vi "whole_setup_control_RT_v1229.vi"() -> ()   [LabVIEW 2021]
uses:
  <vilib>/Utility/file.llb/Read Delimited Spreadsheet (DBL).vi
  <vilib>/FPGAPlugInAG/cRIO-9038/niLvFpga_Open_cRIO-9038.vi
  <vilib>/rvi/interface/common/dynamic/niFpgaDynamicAddResources.vi
  <vilib>/FPGAPlugInAG/Dynamic/niLvFpga_Abort_Dynamic.vi
  <vilib>/FPGAPlugInAG/Dynamic/niLvFpga_Run_Dynamic.vi
  <vilib>/Utility/error.llb/Error Cluster From Error Code.vi
  <vilib>/rvi/errors/niLvFpgaAdjustHostInterfaceError.vi
  <vilib>/Utility/file.llb/Write Delimited Spreadsheet (DBL).vi
  <vilib>/FPGAPlugInAG/Dynamic/niLvFpga_Close_Dynamic.vi
  <vilib>/rvi/interface/nirviOpenFPGA/nirviOpenFPGA.xnode
  FPGA Bitfiles/voltagescopemain_FPGATarget_wholesetupcontro_vB3ODMckxO8.lvbitx
  whole_setup_control_FPGA_v1229.vi
  <vilib>/rvi/interface/nirviMethod/nirviMethod.xnode
  <vilib>/rvi/interface/nirviReadWriteControl/nirviReadWriteControl.xnode
  <vilib>/rvi/interface/nirviCloseFPGA/nirviCloseFPGA.xnode
  <vilib>/rvi/errors/niLvFpgaMergeErrorWithErrorCode.vi
  NiFpgaLv.dll
  <vilib>/rvi/interface/Simulation/niFpgaSimulationCallBeginRW.vi
  <vilib>/FPGAPlugInAG/Dynamic/niLvFpga_StopFifo_Dynamic.vi
  <vilib>/FPGAPlugInAG/Dynamic/niLvFpga_StartFifo_Dynamic.vi
  <vilib>/FPGAPlugInAG/Dynamic/niLvFpga_WriteFifo_Dynamic.vi
  <vilib>/FPGAPlugInAG/Dynamic/niLvFpga_ReadFifo_Dynamic.vi
panel:
  out "Numeric":i32=9
  in  "Signal array length 2":u32=1245
  in  "debug laser delay offset":i32=698
  in  "real laser pulse time (x4us)":i32=10
  in  "laser trigger start points":u32[](array[numeric])=[19, 61, 104, 140, 173, 215, 259, 331, 366, 401, 443, 487, 527, 605, 648, 693, 735, 767, 801, 841, 877, 954, 988, 1021, 1061, 1110, 1153, 1188, 1222, 565]
  in  "update laser triggers RT":bool
  in  "laser ON":bool
  out "Cycle us spent":dbl=4980.0
  in  "Signal array length":u32=1245
  in  "write galvo signal to":path=path "/home/lvuser/zgwang/20231229_4980us_output_signal_corr.dat"
  in  "Write galvo singal to txt RT":bool
  in  "DO 4 laser trigger delay":i32=698
  in  "DO 3 camera trigger delay - DO 4 laser trigger delay":i32=5
  in  "trigger debug?":bool
  in  "debugging and behavior \ncamera trigger delay (loops)":i32
  in  "3F0 freq X":i32=3
  in  "2F0 freq X":i32=5
  in  "camera trigger ON":bool
  in  "Galvo1 corr delay - laser delay":i32=545
  in  "G1 corr amplitude":fxp<+/-,32,16>
  in  "Galvo1 delay":i32=589
  out "ticks spent update":u32=65
  in  "update galvo drive signal RT":bool
  in  "laser delay increament":i32=10
  out "laser delay disp (loops)":i32=1878
  in  "laser delay":i32=118
  out "Loop ticks spent":u32=120
  in  "laser exposure (loops)":i32=10
  in  "Piezo offset":sgl=5.0
  in  "Piezo mag":sgl=2.58
  in  "2F0 amplitude":sgl=0.00255
  in  "3F0 amplitude":sgl=0.0858
  in  "2F0 phase":i32=792
  in  "3F0 phase":i32=555
  in  "Galvo1 offset (mV)":sgl=-448.0
  in  "Galvo1 mag (mV)":sgl=1.0
  out "all rows":dbl[][](array[numeric])
  in  "start output":bool=TRUE
  out "Data transfer finished":bool=TRUE
  in  "output data #":i32=1245
  in  "output loop ticks":u32=160
  in  "stop":bool
  out "array length":i32=1245
  out "Empty Elements Remaining":u32=15139
  out "loop N":i32=10
  in  "file path (dialog if empty)":path=path "/home/lvuser/zgwang/20231229_4980us_output_signal.dat"
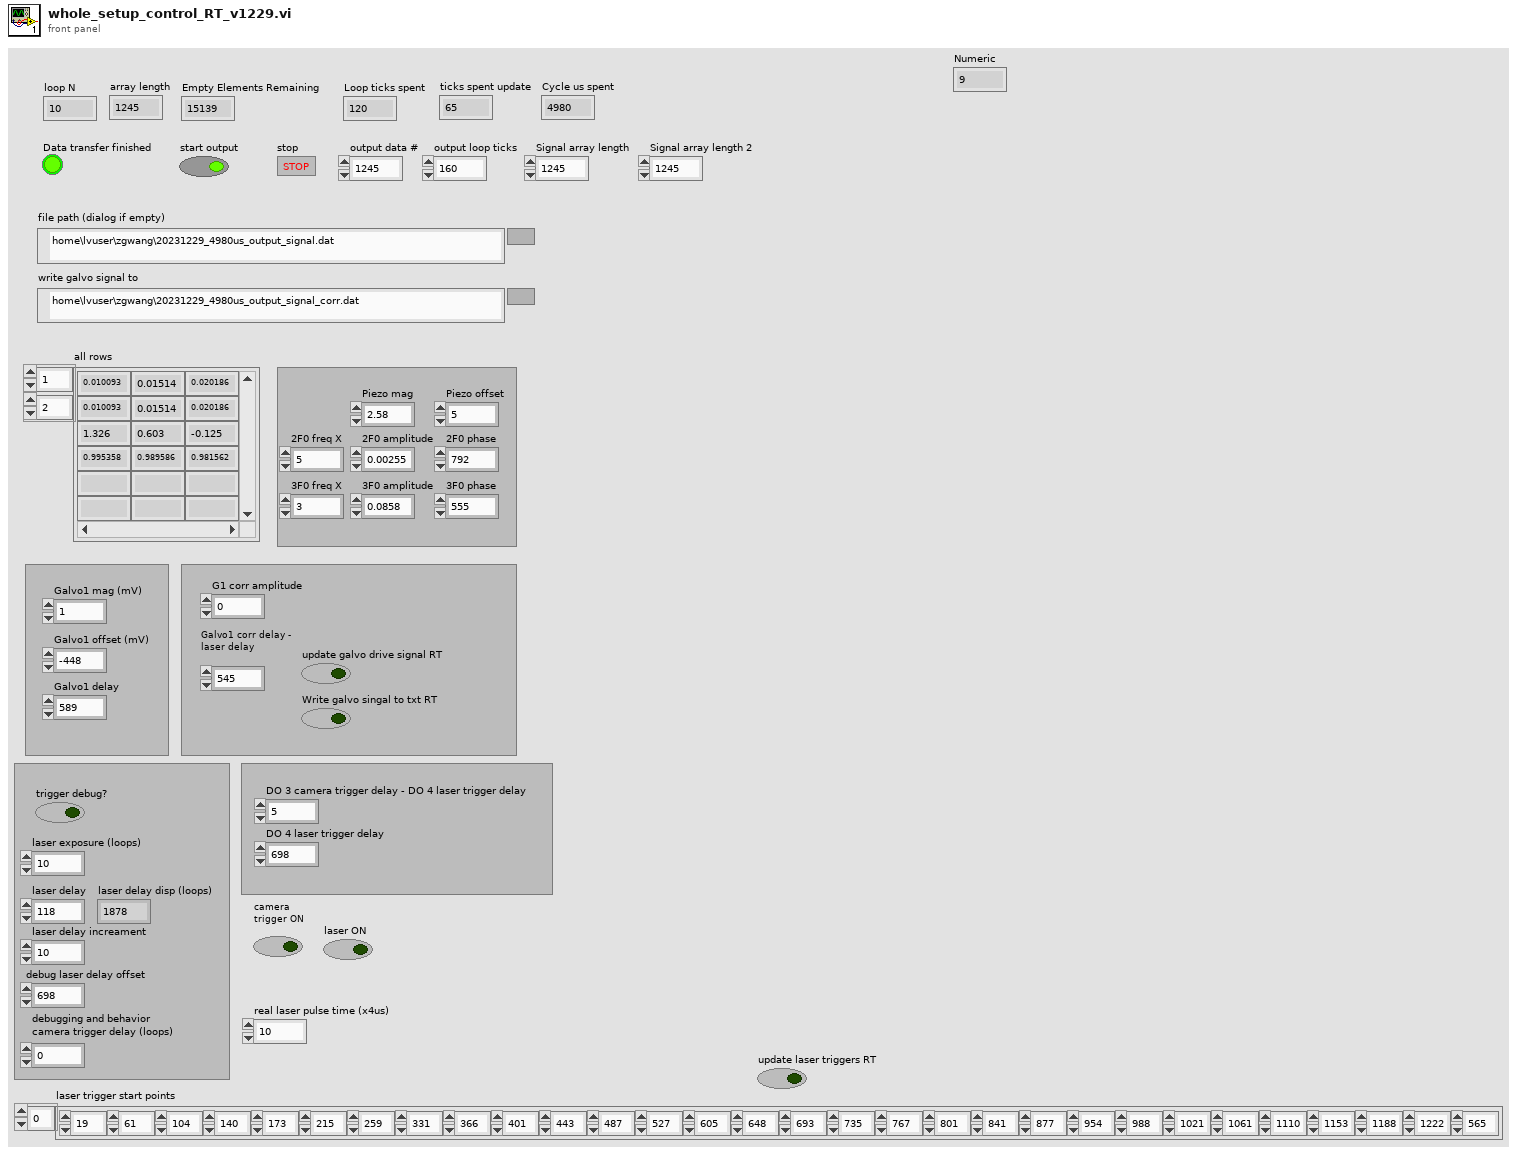
[diagram p1: front panel]
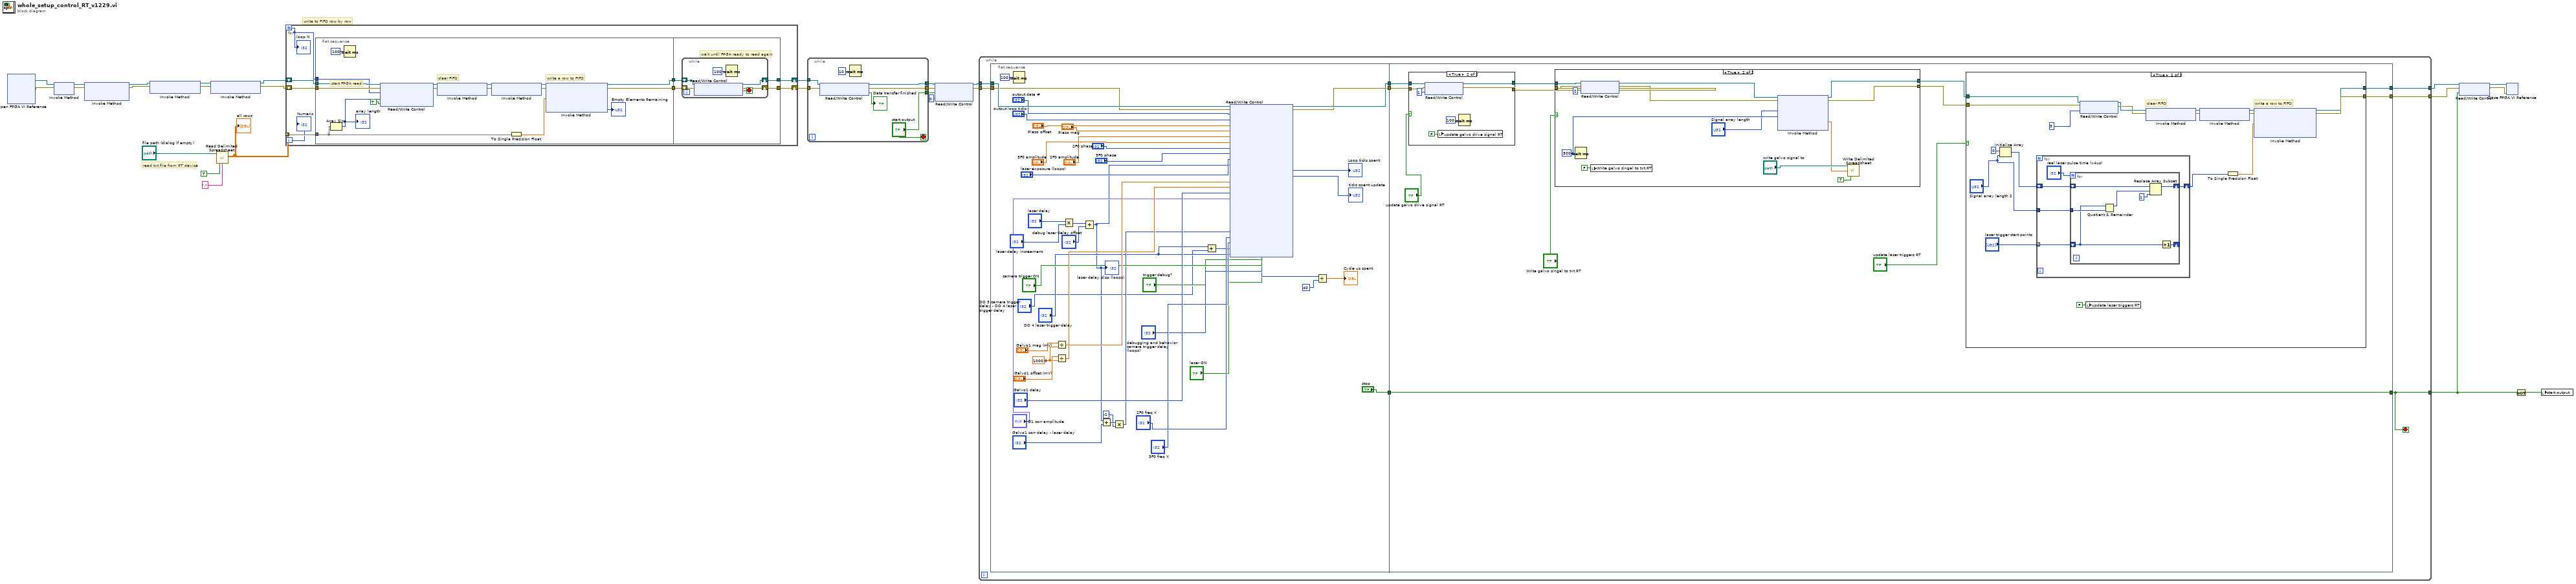
[diagram p0: block diagram]
diagram:
  # "write to FIFO row by row"
  # "read txt file from RT device"
  n1 = xnode "Open FPGA VI Reference"() -> ("FPGA VI Reference Out"=w17:refnum<k20>, "error out"=w14:errorcluster)  [unwired: 2 in]
  n2 = xnode "Invoke Method"("FPGA VI Reference In"=w17, "error in"=w14) -> ("FPGA VI Reference Out"=w16:refnum<k20>, "error out"=w15:errorcluster)
  n3 = xnode "Invoke Method"("FPGA VI Reference In"=w16, "error in"=w15) -> ("FPGA VI Reference Out"=w9:refnum<k20>, "error out"=w8:errorcluster)  [unwired: 1 in]
  n4 = xnode "Invoke Method"("FPGA VI Reference In"=w9, "error in"=w8) -> ("FPGA VI Reference Out"=w11:refnum<k20>, "error out"=w10:errorcluster)
  n5 = xnode "Invoke Method"("FPGA VI Reference In"=w11, "error in"=w10) -> ("FPGA VI Reference Out"=w7:refnum<k20>, "error out"=w6:errorcluster)
  n6 = call-poly <vilib>:"Read Delimited Spreadsheet.vi"("file path (dialog if empty)"="file path (dialog if empty)", "transpose? (F)"=TRUE, "delimiter (\\t)"="," ("delimiter (\\t)")) -> ("all rows"=w25:dbl[][])  [unwired: 7 in, 5 out]
  "all rows" <- w25
  n7 = for {
    N -> [w32]
    tunnel: w25 -> [w37] mode=indexing
    shift-right: [w31] -> w19
    shift-left: w7 -> [w35]
    shift-right: [w30] -> w18
    shift-left: w6 -> [w36]
    i -> [w29]
    n8 = flat-sequence {
      tunnel: w37 -> [w45]
      tunnel: w36 -> [w53]
      tunnel: w35 -> [w52]
      tunnel: [w51] -> w34
      tunnel: [w49] -> w33
      tunnel: w32 -> [w47]
      tunnel: w34 -> [w58]
      tunnel: w33 -> [w57]
      tunnel: [w56] -> w31
      tunnel: [w55] -> w30
      frame #0 {
        # "clear FIFO"
        # "write a row to FIFO"
        # "start FPGA read"
        n9 = Array Size(array=w45) -> (size(s)=w54:i32)
        "array length" <- w54
        n10 = Wait (ms)(milliseconds to wait=u32 100) -> ()  [unwired: 1 out]
        n11 = xnode "Read/Write Control"("FPGA VI Reference In"=w52, "error in"=w53, "data row #"=w47, "array length"=w54, "FPGA start to read FIFO"=TRUE) -> ("FPGA VI Reference Out"=w41:refnum<k20>, "error out"=w40:errorcluster)
        n12 = xnode "Invoke Method"("FPGA VI Reference In"=w41, "error in"=w40) -> ("FPGA VI Reference Out"=w43:refnum<k20>, "error out"=w42:errorcluster)
        n13 = xnode "Invoke Method"("FPGA VI Reference In"=w43, "error in"=w42) -> ("FPGA VI Reference Out"=w39:refnum<k20>, "error out"=w38:errorcluster)
        n14 = To Single Precision Float(number=w45) -> (single precision float=w44:sgl[])
        n15 = xnode "Invoke Method"("FPGA VI Reference In"=w39, "error in"=w38, "Data"=w44) -> ("FPGA VI Reference Out"=w51:refnum<k20>, "error out"=w49:errorcluster, "Empty Elements Remaining"=→"Empty Elements Remaining":u32)  [unwired: 1 in]
      }
      frame #1 {
        # "wait until FPGA ready to read again"
        n16 = while {
          shift-right: [w60] -> w56
          shift-left: w58 -> [w62]
          shift-right: [w59] -> w55
          shift-left: w57 -> [w61]
          stop <- w64 stop-if-true
          n17 = xnode "Read/Write Control"("FPGA VI Reference In"=w62, "error in"=w61) -> ("FPGA VI Reference Out"=w60:refnum<k20>, "error out"=w59:errorcluster, "FPGA finish read row"=w64:bool)
          n18 = Wait (ms)(milliseconds to wait=u32 100) -> ()  [unwired: 1 out]
        }
      }
    }
    "loop N" <- w32
    "Numeric" <- w29
  }
  n19 = while {
    tunnel: ["start output"] -> w24
    tunnel: [w67] -> w21
    tunnel: [w66] -> w20
    tunnel: w19 -> [w69]
    tunnel: w18 -> [w68]
    stop <- "start output" stop-if-true
    n20 = xnode "Read/Write Control"("FPGA VI Reference In"=w69, "error in"=w68) -> ("FPGA VI Reference Out"=w67:refnum<k20>, "error out"=w66:errorcluster, "Data transfer finished"=→"Data transfer finished":bool)
    n21 = Wait (ms)(milliseconds to wait=u32 10) -> ()  [unwired: 1 out]
  }
  n22 = xnode "Read/Write Control"("FPGA VI Reference In"=w21, "error in"=w20, "start output"=w24, "FPGA loop case"=u32 0) -> ("FPGA VI Reference Out"=w23:refnum<k20>, "error out"=w22:errorcluster)
  n23 = while {
    tunnel: w23 -> [w79]
    tunnel: w22 -> [w78]
    tunnel: [w77] -> w12
    tunnel: [w73] -> w2
    tunnel: [w72] -> w1
    stop <- w77 stop-if-true
    n24 = flat-sequence {
      tunnel: w79 -> [w123]
      tunnel: w78 -> [w122]
      tunnel: [w121] -> w76
      tunnel: [w120] -> w75
      tunnel: ["stop"] -> w74
      tunnel: [w136] -> w77
      tunnel: w74 -> [w136]
      tunnel: w75 -> [w131]
      tunnel: w76 -> [w132]
      tunnel: [w126] -> w73
      tunnel: [w125] -> w72
      frame #0 {
        w108 = sgl 1000.0 ("y")
        n25 = Wait (ms)(milliseconds to wait=u32 100) -> ()  [unwired: 1 out]
        n26 = Divide(x="Galvo1 mag (mV)", y=w108) -> (x/y=w103:sgl)
        n27 = Divide(x="Galvo1 offset (mV)", y=w108) -> (x/y=w102:sgl)
        n28 = Multiply(x="laser delay", y="laser delay increament") -> (x*y=w82:i32)
        n29 = Add(x=w82, y="debug laser delay offset") -> (x+y=w80:i32)
        "laser delay disp (loops)" <- w80
        n30 = Add(x=w80, y="Galvo1 corr delay - laser delay") -> (x+y=w99:i32)
        n31 = Multiply(x=w99, y=-1) -> (x*y=w92:i32)
        n32 = Add(x="DO 4 laser trigger delay", y="DO 3 camera trigger delay - DO 4 laser trigger delay") -> (x+y=w83:i32)
        n33 = xnode "Read/Write Control"("FPGA VI Reference In"=w123, "error in"=w122, "output data #"="output data #", "output loop ticks"="output loop ticks", "Piezo offset"="Piezo offset", "Piezo mag"="Piezo mag", "2F0 amplitude"="2F0 amplitude", "3F0 amplitude"="3F0 amplitude", "2F0 phase relative to F0"="2F0 phase", "3F0 phase relative to F0"="3F0 phase", "laser exposure (loops)"="laser exposure (loops)", "laser delay (loops)"=w80, "Galvo1 mag"=w103, "Galvo1 offset"=w102, "Galvo1 delay"="Galvo1 delay", "G1 corr amplitude"="G1 corr amplitude", "Galvo1 corr delay"=w92, "2F0 freq X"="2F0 freq X", "3F0 freq X"="3F0 freq X", "DO 3 delay"=w83, "DO 4 delay"="DO 4 laser trigger delay", "trigger debug?"="trigger debug?", "camera trigger ON"="camera trigger ON", "camera trigger delay (loops)"="debugging and behavior \ncamera trigger delay (loops)", "laser ON"="laser ON") -> ("FPGA VI Reference Out"=w121:refnum<k20>, "error out"=w120:errorcluster, "Loop ticks spent"=→"Loop ticks spent":u32, "ticks spent update"=→"ticks spent update":u32, "Cycle tick spent"=w89:u32)
        n34 = Divide(x=w89, y=u32 40) -> (x/y=→"Cycle us spent":dbl)
      }
      frame #1 {
        n35 = case shown="True" "update galvo drive signal RT" {
          tunnel: w132 -> [w169 w177]
          tunnel: [w169 w176] -> w134
          tunnel: [w170 w175] -> w133
          tunnel: w131 -> [w170 w174]
          frame False {
          }
          frame True {
            n36 = xnode "Read/Write Control"("FPGA VI Reference In"=w177, "error in"=w174, "FPGA loop case"=u32 1) -> ("FPGA VI Reference Out"=w176:refnum<k20>, "error out"=w175:errorcluster)
            n37 = local write "update galvo drive signal RT"(FALSE ("update galvo drive signal RT")) -> ()
            n38 = Wait (ms)(milliseconds to wait=u32 100) -> ()  [unwired: 1 out]
          }
        }
        n39 = case shown="True" "Write galvo singal to txt RT" {
          tunnel: w134 -> [w179 w192]
          tunnel: w133 -> [w178 w191]
          tunnel: [w179 w186] -> w128
          tunnel: [w178 w185] -> w127
          frame False {
          }
          frame True {
            w184 = u32 500 ("milliseconds to wait")
            n40 = Wait (ms)(milliseconds to wait=w184) -> ()  [unwired: 1 out]
            n41 = xnode "Read/Write Control"("FPGA VI Reference In"=w192, "error in"=w191, "FPGA loop case"=u32 2) -> ("FPGA VI Reference Out"=w188:refnum<k20>, "error out"=w187:errorcluster)
            n42 = local write "Write galvo singal to txt RT"(FALSE ("Write galvo singal to txt RT")) -> ()
            n43 = xnode "Invoke Method"("FPGA VI Reference In"=w188, "error in"=w187, "Number of Elements"="Signal array length", "Timeout (ms)"=w184) -> ("FPGA VI Reference Out"=w186:refnum<k20>, "error out"=w185:errorcluster, "Data"=w182:sgl[])  [unwired: 1 out]
            n44 = call-poly <vilib>:"Write Delimited Spreadsheet.vi"("file path (dialog if empty)"="write galvo signal to", "1D data"=w182, "transpose? (no:F)"=TRUE) -> ()  [unwired: 11 in, 2 out]
          }
        }
        n45 = case shown="True" "update laser triggers RT" {
          tunnel: w128 -> [w137 w144]
          tunnel: w127 -> [w138 w142]
          tunnel: [w138 w147] -> w125
          tunnel: [w137 w146] -> w126
          frame False {
          }
          frame True {
            # "clear FIFO"
            # "write a row to FIFO"
            n46 = Initialize Array(u32 0 ("element"), "Signal array length 2") -> (w154:u32[])
            n47 = for {
              tunnel: "laser trigger start points" -> [w160] mode=indexing
              shift-right: [w159] -> w148
              shift-left: w154 -> [w161]
              tunnel: "Signal array length 2" -> [w157]
              n48 = for {
                N: "real laser pulse time (x4us)" -> [_]
                shift-right: [w165] -> w159
                shift-left: w161 -> [w168]
                shift-right: [w166] -> _
                shift-left: w160 -> [w163]
                tunnel: w157 -> [w164]
                n49 = Quotient & Remainder(x=w163, y=w164) -> (x-y*floor(x/y)=w162:u32)  [unwired: 1 out]
                n50 = Replace Array Subset(array=w168, new element=u32 1 ("new element/subarray"), index=w162) -> (w165:u32[])
                n51 = Increment(x=w163) -> (x+1=w166:u32)
              }
            }
            n52 = xnode "Read/Write Control"("FPGA VI Reference In"=w144, "error in"=w142, "FPGA loop case"=u32 3) -> ("FPGA VI Reference Out"=w143:refnum<k20>, "error out"=w141:errorcluster)
            n53 = local write "update laser triggers RT"(FALSE ("update laser triggers RT")) -> ()
            n54 = xnode "Invoke Method"("FPGA VI Reference In"=w143, "error in"=w141) -> ("FPGA VI Reference Out"=w153:refnum<k20>, "error out"=w152:errorcluster)
            n55 = xnode "Invoke Method"("FPGA VI Reference In"=w153, "error in"=w152) -> ("FPGA VI Reference Out"=w151:refnum<k20>, "error out"=w150:errorcluster)
            n56 = To Single Precision Float(number=w148) -> (single precision float=w149:sgl[])
            n57 = xnode "Invoke Method"("FPGA VI Reference In"=w151, "error in"=w150, "Data"=w149) -> ("FPGA VI Reference Out"=w146:refnum<k20>, "error out"=w147:errorcluster)  [unwired: 1 in, 1 out]
          }
        }
      }
    }
  }
  n58 = xnode "Read/Write Control"("FPGA VI Reference In"=w2, "error in"=w1, "stop output"=w12) -> ("FPGA VI Reference Out"=w5:refnum<k20>, "error out"=w4:errorcluster)
  n59 = xnode "Close FPGA VI Reference"("FPGA VI Reference In"=w5, "error in"=w4) -> ()  [unwired: 1 out]
  n60 = Not(x=w12) -> (.not. x?=w13:bool)
  n61 = local write "start output"(w13) -> ()
